vi "LCR_Init.vi"(8 "error in (no error)":errorcluster, 11 "LCRControl in":refnum<class "LCRControl.lvclass">) -> (0 "error out":errorcluster, 3 "LCRControl out":refnum<class "LCRControl.lvclass">)   [LabVIEW 2013, in "LCRControl.lvclass"]
uses:
  LCRControl.lvclass
  InstrControl.lvclass
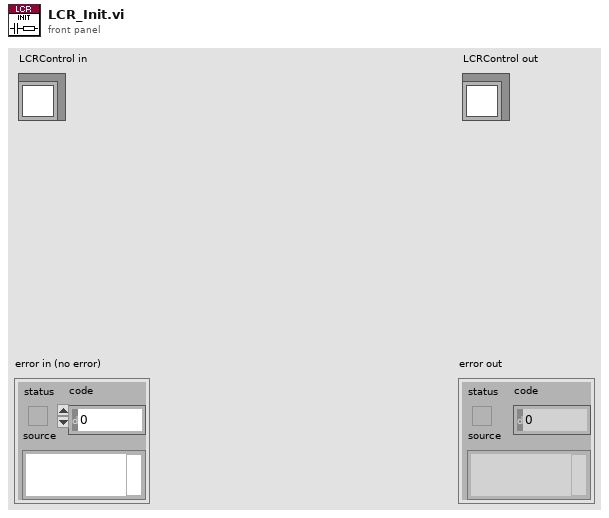
[diagram p1: front panel]
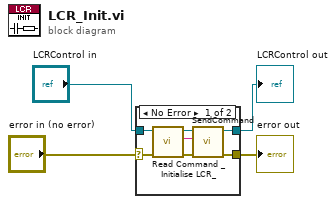
[diagram p0: block diagram]
diagram:
  n1 = case shown="No Error" "error in (no error)" {
    selector: "error in (no error)" -> [w5 w13]
    tunnel: [w7 w13] -> w3
    tunnel: [w11 w12] -> w1
    tunnel: "LCRControl in" -> [w6 w12]
    frame No Error {
      n2 = call-dynamic "Read Command _Initialise LCR_.vi"("error in (no error)"=w5, "LCRControl in"=w6) -> ("error out"=w8:errorcluster, "Command \"Initialise LCR\""=w9:string, "LCRControl out"=w10:refnum<class "LCRControl.lvclass">)  [unwired: 7 in]
      n3 = call "SendCommand.vi"("error in (no error)"=w8, "Command string"=w9, "InstControl in"=w10) -> ("error out"=w7:errorcluster, "InstControl out"=w11:refnum<class "LCRControl.lvclass">)  [unwired: 7 in]
    }
    frame Error {
    }
  }
  "error out" <- w3
  "LCRControl out" <- w1
